vi "RandomPointGenerator.vi"(9 "Field defense":dbl[](array[numeric]), 10 "IA State Input":T1) -> (2 "Point Ally Field":dbl[](array[numeric]))   [LabVIEW 2017]
uses:
  Core/AI Input.ctl
  Core/AI Robot.ctl
  Intel/Functions Enum.ctl
  Intel/AttackerStates.ctl
  Path Planning/RRT/PathDests.ctl
  Path Planning/RRT/PathDest.ctl
  Core/AI Ball.ctl
  Core/Field Size.ctl
  Core/AI Judge.ctl
  Intel/Command Enum.ctl
  Util/Events/Events.ctl
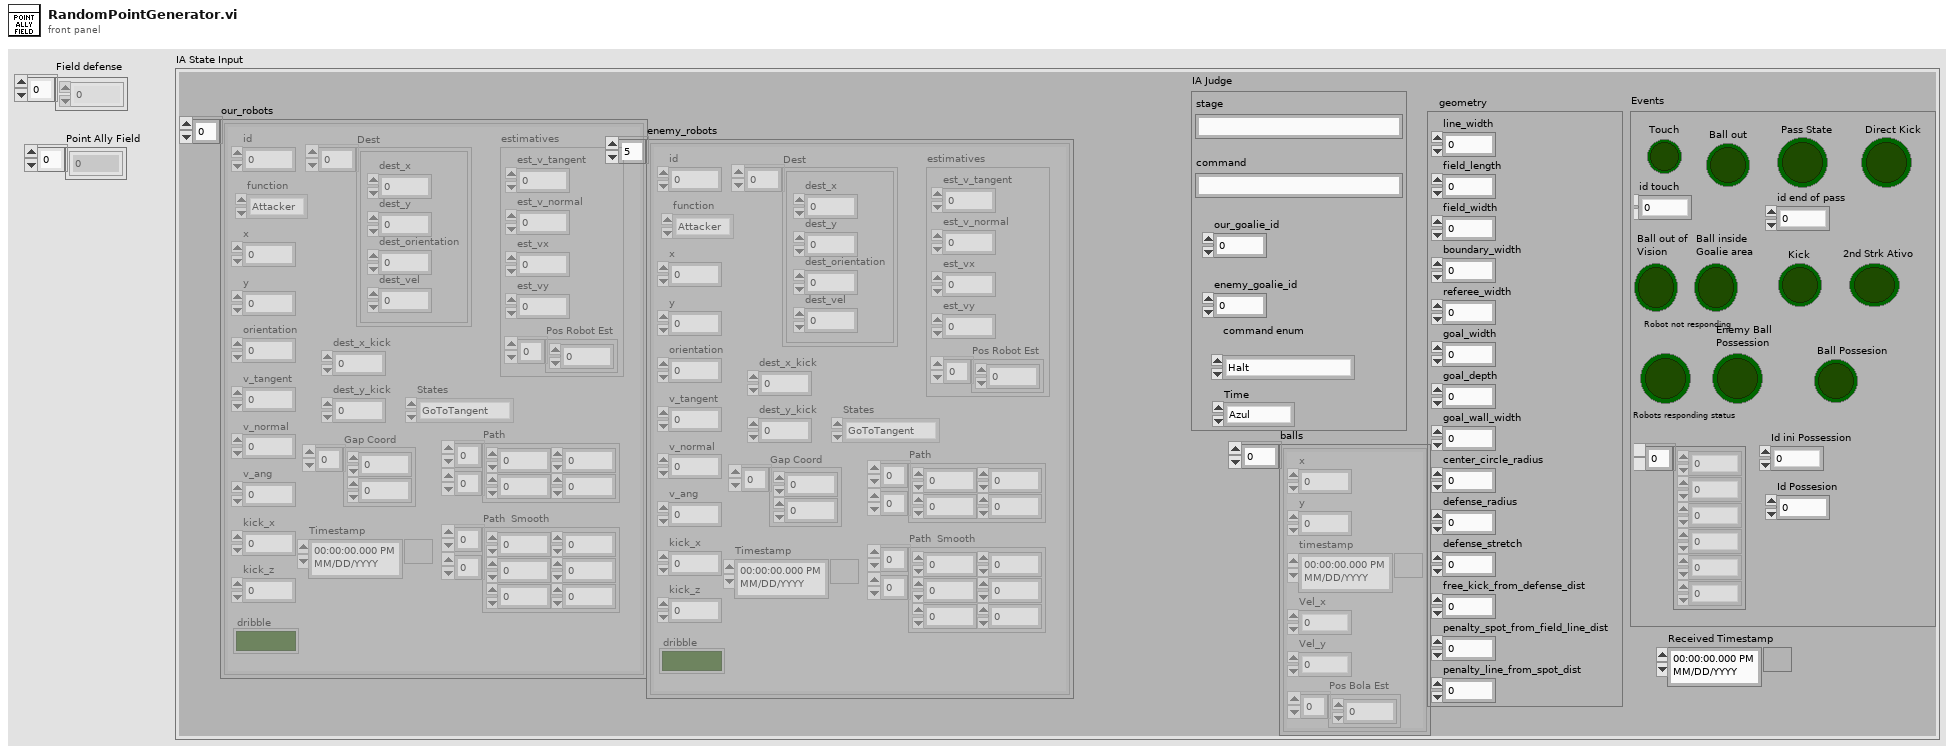
[diagram p1: front panel]
types:
  T1 = typedef "AI Input.ctl" = cluster{"our_robots":T2[], "enemy_robots":T2[], "balls":T7[], "geometry":T8, "IA Judge":T9, "Received Timestamp":timestamp, "Events":T11}
  T2 = typedef "AI Robot.ctl" = cluster{"id":u32, "function":T3, "x":dbl, "y":dbl, "orientation":dbl, "v_tangent":dbl, "v_normal":dbl, "v_ang":dbl, "kick_x":dbl, "kick_z":dbl, "dribble":bool, "Timestamp":timestamp, "estimatives":cluster{"est_v_tangent":dbl, "est_v_normal":dbl, "est_vx":dbl, "est_vy":dbl, "Pos Robot Est":dbl[]}, "dest_x_kick":dbl, "dest_y_kick":dbl, "Gap Coord":dbl[], "States":T4, "Path ":dbl[][], "Path  Smooth":dbl[][], "Dest":T5}
  T3 = typedef "Functions Enum.ctl" = enum16{"2nd Striker", "Attacker", "Goalie", "Defender", "Striker", "Goto 0", "Dummy", "Kicker", "ZigZag 0", "ZigZag 1", "ZigZag 2", "ZigZag 3", "ZigZag 4", "ZigZag 5", "ZigZag 6", "ZigZag 7", "ZigZag 8", ""}
  T4 = typedef "AttackerStates.ctl" = enum16{"Pass", "GoToTangent", "BallGetting", "GoToKick", ""}
  T5 = typedef "PathDests.ctl" = T6[]
  T6 = typedef "PathDest.ctl" = cluster{"dest_x":dbl, "dest_y":dbl, "dest_orientation":dbl, "dest_vel":dbl}
  T7 = typedef "AI Ball.ctl" = cluster{"x":dbl, "y":dbl, "timestamp":timestamp, "Vel_x":dbl, "Vel_y":dbl, "Pos Bola Est":dbl[]}
  T8 = typedef "Field Size.ctl" = cluster{"line_width":u32, "field_length":u32, "field_width":u32, "boundary_width":u32, "referee_width":u32, "goal_width":u32, "goal_depth":u32, "goal_wall_width":u32, "center_circle_radius":u32, "defense_radius":u32, "defense_stretch":u32, "free_kick_from_defense_dist":u32, "penalty_spot_from_field_line_dist":u32, "penalty_line_from_spot_dist":u32}
  T9 = typedef "AI Judge.ctl" = cluster{"stage":string, "command":string, "our_goalie_id":dbl, "enemy_goalie_id":dbl, "command enum":T10, "Time":enum16{"Azul", "Amarelo"}}
  T10 = typedef "Command Enum.ctl" = enum16{"Halt", "Stop", "Force Start", "PKA Normal Start", "Prepare Kickoff Ally", "PKE Normal Start", "Prepare Kickoff Enemy", "Prepare Penalty Ally", "PPA Normal Start", "Prepare Penalty Enemy", "PPE Normal Start", "Direct Free Enemy", "Direct Free Ally", "Indirect Free Enemy", "Indirect Free Ally", "Timeout Enemy", "Timeout Ally", "Goal Enemy", "Goal Ally", "Ball Placement Enemy", "Ball Placement Ally", "Normal Half Time", "Extra Time Break", "Extra Half Time", "None", "Post Game"}
  T11 = typedef "Events.ctl" = cluster{"Touch":bool, "Ball out":bool, "id touch":dbl, "Ball out of \nVision":bool, "Ball inside \nGoalie area":bool, "Robot not responding":bool, "Robots responding status":dbl[], "Enemy Ball \nPossession":bool, "Pass State":bool, "id end of pass":dbl, "Kick":bool, "Id ini Possession":dbl, "Ball Possesion":bool, "Id Possesion":dbl, "Direct Kick":bool, "2nd Strk Ativo":bool}
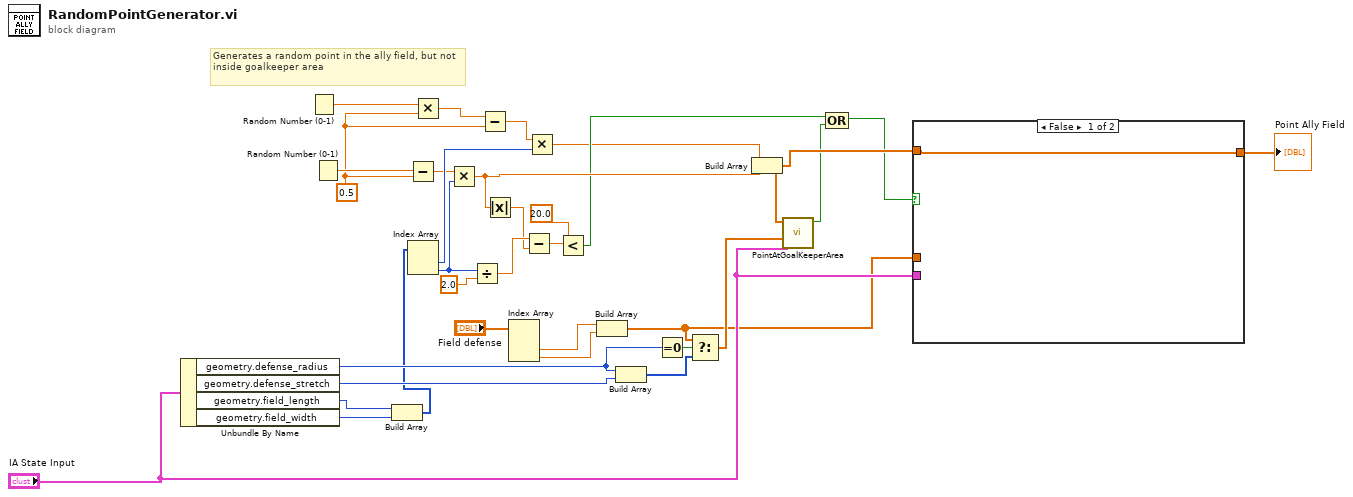
[diagram p0: block diagram]
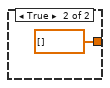
[diagram p2: hidden frame]
diagram:
  w28 = 0.5 ("y")
  # "Generates a random point in the ally field, but not inside goalkeeper area"
  n1 = Unbundle By Name("IA State Input") -> ("geometry.defense_radius"=w11:u32, "geometry.defense_stretch"=w13:u32, "geometry.field_length"=w1:u32, "geometry.field_width"=w8:u32)
  n2 = Random Number (0-1)() -> (number: 0 to 1=w30:dbl)
  n3 = Random Number (0-1)() -> (number: 0 to 1=w31:dbl)
  n4 = Build Array(w1, w8) -> (w7:u32[])
  n5 = Subtract(x=w31, y=w28) -> (x-y=w32:dbl)
  n6 = Index Array(array=w7) -> (element #1=w33:u32, element #2=w24:u32)  [unwired: 2 in]
  n7 = Multiply(x=w30, y=w28) -> (x*y=w29:dbl)
  n8 = Multiply(x=w32, y=w24) -> (x*y=w22:dbl)
  n9 = Divide(x=w24, y=2.0) -> (x/y=w21:dbl)
  n10 = Subtract(x=w29, y=w28) -> (x-y=w27:dbl)
  n11 = Absolute Value(x=w22) -> (abs(x)=w20:dbl)
  n12 = Index Array(array="Field defense") -> (element #2=w5:dbl, element #3=w4:dbl)  [unwired: 3 in, 1 out]
  n13 = Subtract(x=w21, y=w20) -> (x-y=w19:dbl)
  n14 = Multiply(x=w27, y=w33) -> (x*y=w2:dbl)
  n15 = Less?(x=w19, y=20.0) -> (x < y?=w16:bool)
  n16 = Build Array(w5, w4) -> (w3:dbl[])
  n17 = Build Array(w11, w13) -> (w10:u32[])
  n18 = Equal To 0?(x=w11) -> (x = 0?=w12:bool)
  n19 = Select(t=w3, s=w12, f=w10) -> (s? t:f=w9:dbl[])
  n20 = Build Array(w2, w22) -> (w26:dbl[])
  n21 = call "PointAtGoalKeeperArea.vi"("Field defense"=w9, "IA State Input"="IA State Input", "Array"=w26) -> ("Point inside goalkeeper area ?"=w17:bool)  [unwired: 8 in]
  n22 = Compound Arithmetic op=OR(w16, w17) -> (w15:bool)
  n23 = case shown="False" w15 {
    tunnel: [w34 dbl[] []] -> w25
    tunnel: w26 -> [w34 _]
    tunnel: "IA State Input" -> [_ _]
    tunnel: w3 -> [_ _]
    frame False {
    }
    frame True {
    }
  }
  "Point Ally Field" <- w25
